vi "Keyence.Tune.vi"(0 "cID in":refnum<k5>, 11 "error in":errorcluster, 12 "Timeout [ms] (1000)":i32=1000) -> (4 "cID out":refnum<k5>, 6 "OK?":bool, 8 "Response":string, 15 "error out":errorcluster)   [LabVIEW 2015]
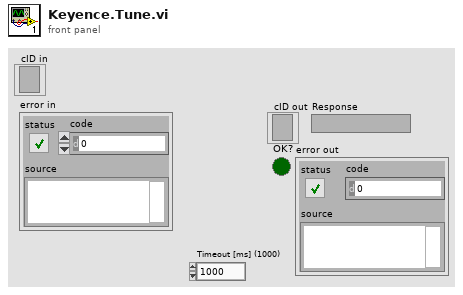
[diagram p1: front panel]
types:
  T1 = enum16{"Standard", "Buffered", "CRLF", "Immediate"}
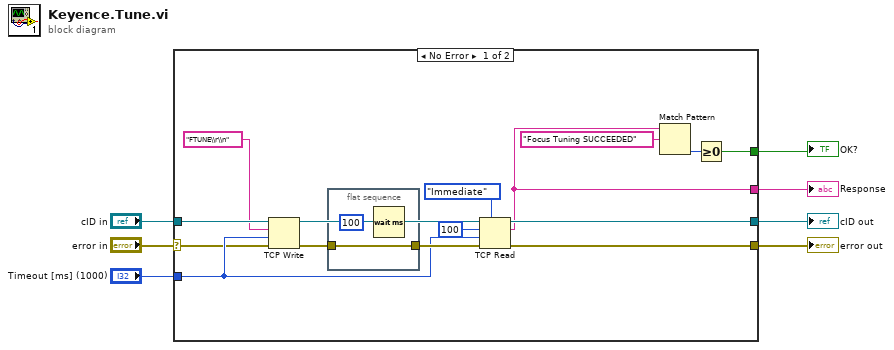
[diagram p0: block diagram]
diagram:
  n1 = case shown="No Error" "error in" {
    selector: "error in" -> [w17 w25]
    tunnel: "Timeout [ms] (1000)" -> [w19 _]
    tunnel: "cID in" -> [w18 w26]
    tunnel: [w11 w26] -> w4
    tunnel: [w12 w25] -> w3
    tunnel: [w10 _] -> w2
    tunnel: [w9 _] -> w1
    frame No Error {
      n2 = TCP Write(connection ID=w18, data in="FTUNE\\r\\n", error in (no error)=w17, 9:w19) -> (connection ID out=w20:refnum<k5>, error out=w22:errorcluster)  [unwired: 1 out]
      n3 = flat-sequence {
        tunnel: w22 -> [w24]
        tunnel: [w24] -> w21
        frame #0 {
          n4 = Wait (ms)(milliseconds to wait=u32 100) -> ()  [unwired: 1 out]
        }
      }
      n5 = TCP Read(connection ID=w20, bytes to read=100, error in (no error)=w21, 7:T1."Immediate" ("mode (standard)"), 9:w19) -> (connection ID out=w11:refnum<k5>, data out=w9:string, error out=w12:errorcluster)
      n6 = Match Pattern(string=w9, regular expression="Focus Tuning SUCCEEDED") -> (offset past match=w13:i32)  [unwired: 1 in, 3 out]
      n7 = Greater Or Equal To 0?(x=w13) -> (x >= 0?=w10:bool)
    }
    frame Error {
    }
  }
  "cID out" <- w4
  "Response" <- w1
  "OK?" <- w2
  "error out" <- w3
